vi "GetParam.vi"(8 "error in (no error)":errorcluster caption="entrée d'erreur (pas d'erreur)", 11 "Pairwise_kernels.lvclass":refnum<class "Pairwise_kernels.lvclass">) -> (0 "error out":errorcluster caption="sortie d'erreur", 2 "pairwise_kernels":T1={"metric "="linear", "filter_params"=FALSE, "n_jobs"="None"}, 3 "Pairwise_kernels.lvclass":refnum<class "Pairwise_kernels.lvclass">)   [LabVIEW 2020, in "Pairwise_kernels.lvclass"]
doc: "Get Parameters"
uses:
  Pairwise_kernels.lvclass
  Pairwise_kernels.lvclass/Pairwise_kernels.ctl
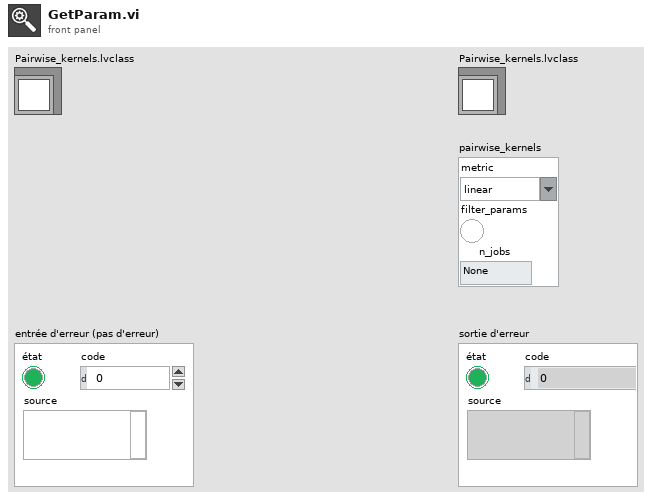
[diagram p1: front panel]
types:
  T1 = cluster{"metric ":string, "filter_params":bool, "n_jobs":string}
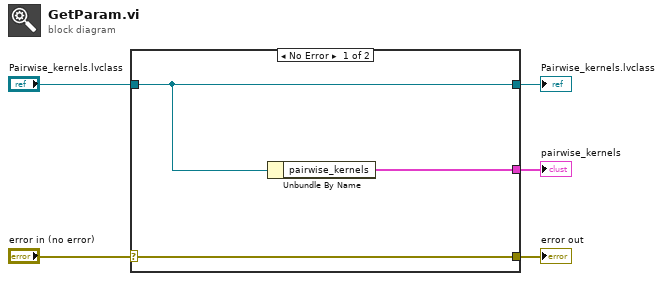
[diagram p0: block diagram]
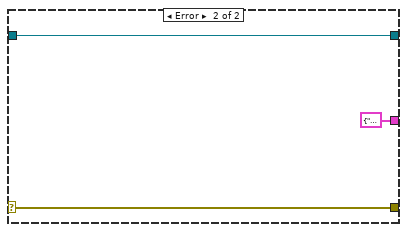
[diagram p2: hidden frame]
diagram:
  n1 = case shown="No Error" "error in (no error)" {
    selector: "error in (no error)" -> [w8 w10]
    tunnel: [w8 w10] -> w4
    tunnel: [w7 w11] -> w2
    tunnel: "Pairwise_kernels.lvclass" -> [w7 w11]
    tunnel: [w6 T1 {"metric "="", "filter_params"=FALSE, "n_jobs"=""} ("pairwise_kernels")] -> w1
    frame No Error {
      n2 = Unbundle By Name(w7) -> ("pairwise_kernels"=w6:T1)
    }
    frame Error {
    }
  }
  "error out" <- w4
  "Pairwise_kernels.lvclass" <- w2
  "pairwise_kernels" <- w1
